vi "MatlabPathClear.vi"(8 "error in":errorcluster, 11 "Path":path) -> (0 "error out":errorcluster)   [LabVIEW 2015]
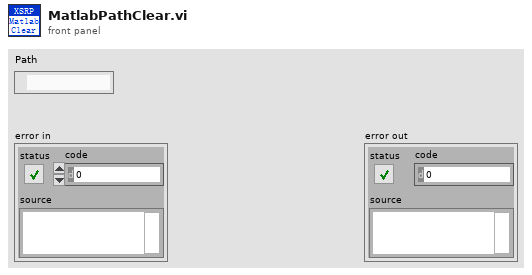
[diagram p1: front panel]
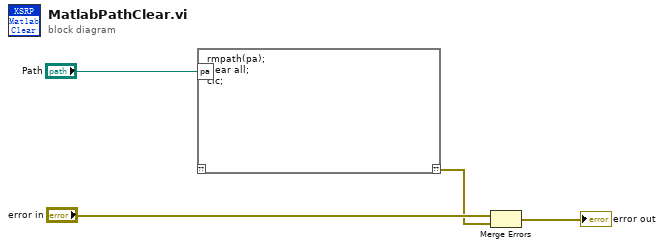
[diagram p0: block diagram]
diagram:
  n1 = script code="rmpath(pa);\nclear all;\nclc;"("pa"="Path") -> ("??"=w2:errorcluster)  [unwired: 1 out]
  n2 = Merge Errors("error in", w2) -> (→"error out":errorcluster)
